vi "writeDrive.vi"(8 "error in (no error)":errorcluster, 9 "Pod Number":i32, 10 "Drive":T2, 11 "Refnum in":T1) -> (0 "error out":errorcluster, 3 "Refnum in 2":T1)   [LabVIEW 2014]
uses:
  <vilib>/Utility/config.llb/Config Data RefNum.ctl
  <vilib>/Utility/config.llb/Write Key (Double).vi
  <vilib>/Utility/config.llb/Write Key (String).vi
  <vilib>/Utility/config.llb/Write Key (I32).vi
  <vilib>/Utility/config.llb/Write Key (Boolean).vi
  <vilib>/Utility/config.llb/NI_LVConfig.lvlib
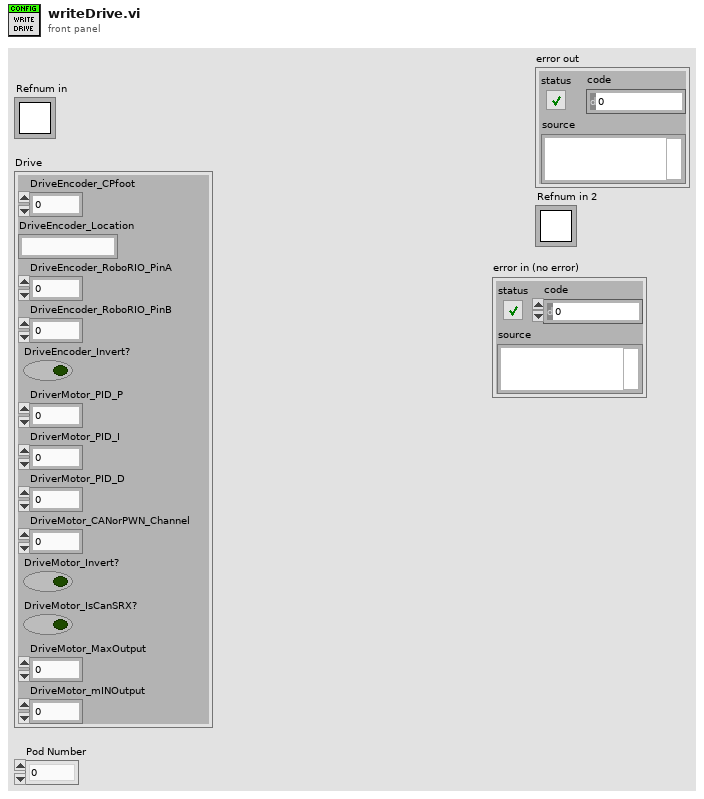
[diagram p1: front panel]
types:
  T1 = typedef "NI_LVConfig.lvlib/Config Data RefNum.ctl" = refnum<k1>
  T2 = cluster{"DriveEncoder_CPfoot":dbl, "DriveEncoder_Location":string, "DriveEncoder_RoboRIO_PinA":i32, "DriveEncoder_RoboRIO_PinB":i32, "DriveEncoder_Invert?":bool, "DriverMotor_PID_P":dbl, "DriverMotor_PID_I":dbl, "DriverMotor_PID_D":dbl, "DriveMotor_CANorPWN_Channel":i32, "DriveMotor_Invert?":bool, "DriveMotor_IsCanSRX?":bool, "DriveMotor_MaxOutput":dbl, "DriveMotor_mINOutput":dbl}
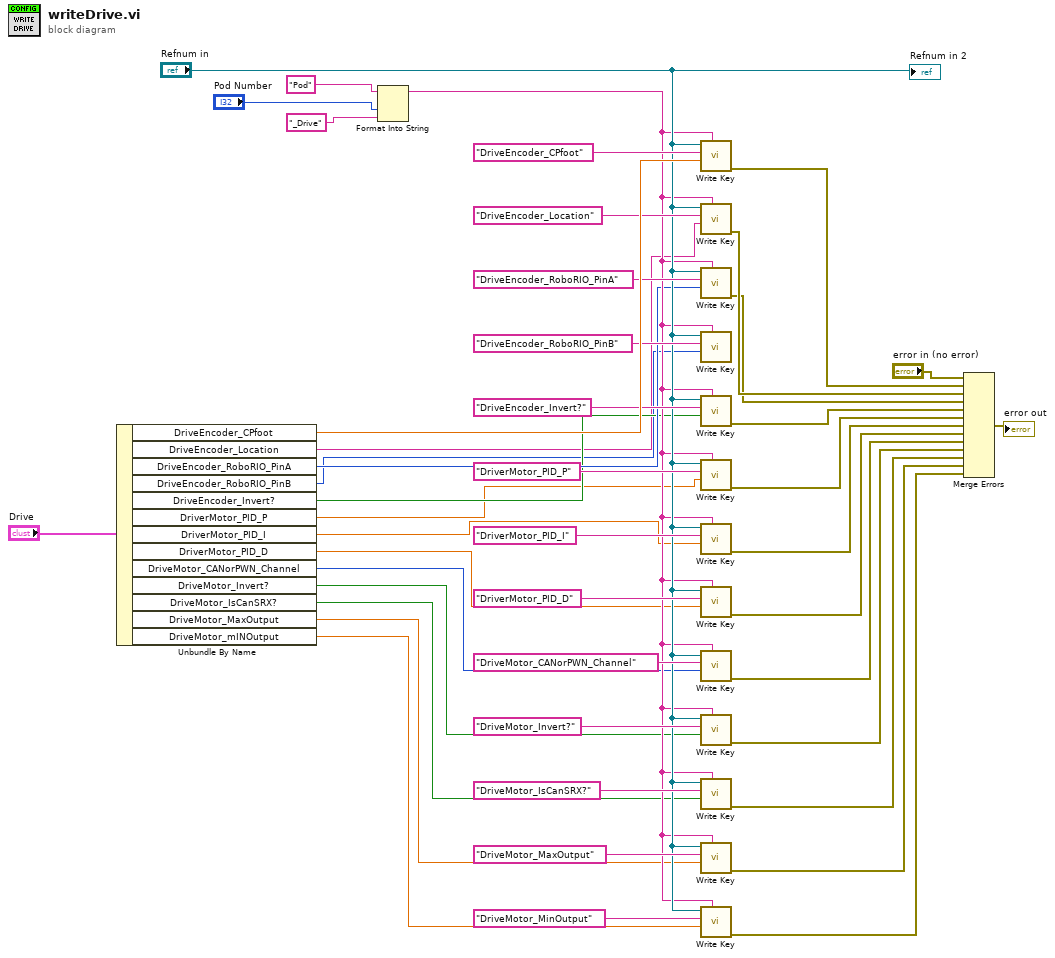
[diagram p0: block diagram]
diagram:
  n1 = Unbundle By Name("Drive") -> ("DriveEncoder_CPfoot"=w46:dbl, "DriveEncoder_Location"=w15:string, "DriveEncoder_RoboRIO_PinA"=w26:i32, "DriveEncoder_RoboRIO_PinB"=w16:i32, "DriveEncoder_Invert?"=w25:bool, "DriverMotor_PID_P"=w24:dbl, "DriverMotor_PID_I"=w17:dbl, "DriverMotor_PID_D"=w18:dbl, "DriveMotor_CANorPWN_Channel"=w23:i32, "DriveMotor_Invert?"=w19:bool, "DriveMotor_IsCanSRX?"=w22:bool, "DriveMotor_MaxOutput"=w21:dbl, "DriveMotor_mINOutput"=w20:dbl)
  n2 = Format Into String(initial string="Pod", "Pod Number", "_Drive") -> (resulting string=w27:string)  [unwired: 2 in, 1 out]
  n3 = call-poly <vilib>:"Write Key.vi"("section"=w27, "value"=w46, "key"="DriveEncoder_CPfoot", "refnum"="Refnum in") -> ("error out"=w14:errorcluster)  [unwired: 5 in, 2 out]
  n4 = call-poly <vilib>:"Write Key.vi"("section"=w27, "value"=w15, "key"="DriveEncoder_Location", "refnum"="Refnum in") -> ("error out"=w13:errorcluster)  [unwired: 5 in, 2 out]
  n5 = call-poly <vilib>:"Write Key.vi"("section"=w27, "value"=w26, "key"="DriveEncoder_RoboRIO_PinA", "refnum"="Refnum in") -> ("error out"=w12:errorcluster)  [unwired: 5 in, 2 out]
  n6 = call-poly <vilib>:"Write Key.vi"("section"=w27, "value"=w16, "key"="DriveEncoder_RoboRIO_PinB", "refnum"="Refnum in") -> ()  [unwired: 5 in, 3 out]
  n7 = call-poly <vilib>:"Write Key.vi"("section"=w27, "value"=w25, "key"="DriveEncoder_Invert?", "refnum"="Refnum in") -> ("error out"=w11:errorcluster)  [unwired: 5 in, 2 out]
  n8 = call-poly <vilib>:"Write Key.vi"("section"=w27, "value"=w24, "key"="DriverMotor_PID_P", "refnum"="Refnum in") -> ("error out"=w10:errorcluster)  [unwired: 5 in, 2 out]
  n9 = call-poly <vilib>:"Write Key.vi"("section"=w27, "value"=w17, "key"="DriverMotor_PID_I", "refnum"="Refnum in") -> ("error out"=w9:errorcluster)  [unwired: 5 in, 2 out]
  n10 = call-poly <vilib>:"Write Key.vi"("section"=w27, "value"=w18, "key"="DriverMotor_PID_D", "refnum"="Refnum in") -> ("error out"=w8:errorcluster)  [unwired: 5 in, 2 out]
  n11 = call-poly <vilib>:"Write Key.vi"("section"=w27, "value"=w23, "key"="DriveMotor_CANorPWN_Channel", "refnum"="Refnum in") -> ("error out"=w7:errorcluster)  [unwired: 5 in, 2 out]
  n12 = call-poly <vilib>:"Write Key.vi"("section"=w27, "value"=w19, "key"="DriveMotor_Invert?", "refnum"="Refnum in") -> ("error out"=w6:errorcluster)  [unwired: 5 in, 2 out]
  n13 = call-poly <vilib>:"Write Key.vi"("section"=w27, "value"=w22, "key"="DriveMotor_IsCanSRX?", "refnum"="Refnum in") -> ("error out"=w5:errorcluster)  [unwired: 5 in, 2 out]
  n14 = call-poly <vilib>:"Write Key.vi"("section"=w27, "value"=w21, "key"="DriveMotor_MaxOutput", "refnum"="Refnum in") -> ("error out"=w4:errorcluster)  [unwired: 5 in, 2 out]
  n15 = call-poly <vilib>:"Write Key.vi"("section"=w27, "value"=w20, "key"="DriveMotor_MinOutput", "refnum"="Refnum in") -> ("error out"=w3:errorcluster)  [unwired: 5 in, 2 out]
  n16 = Merge Errors("error in (no error)", w14, w13, w12, w11, w10, w9, w8, w7, w6, w5, w4, w3) -> (→"error out":errorcluster)
  "Refnum in 2" <- "Refnum in"
